vi "Shutter Tuning Interface.vi"(4 "Legacy thrsh (nA)":sgl=0.005 min=0 step=0.0005, 6 "Damped thrsh (nA)":sgl=0.004999995 min=0 step=0.0005, 7 "Shutter Drive":tag="Log/ao0", 10 "Damping":bool=TRUE, 11 "configuration file path":path=path "D:/3D FIB-SEM Files/Jeiss.ini") -> (3 "SEM shutter status":string, 5 "Damping out":bool)   [LabVIEW 2018]
panel:
  out "Specimen I Graph":dbl[](graph)
  in  "Legacy Pulse (ms)":u16=1000
  in  "Pulse Times":u16[][](array[numeric])
  in  "Restore Defaults":bool
  in  "Read from INI":bool
  in  "Write INI":bool
  out "SDev":sgl format="%.4f"
  in  "OPEN-CLOSE":bool
  in  "stop":bool
  # "Pulse Time Fuctions: \n  DeStick, Start, Swing, Brake, Wait, Retain, zeros."
  # "(Close)"
  # "(Open)"
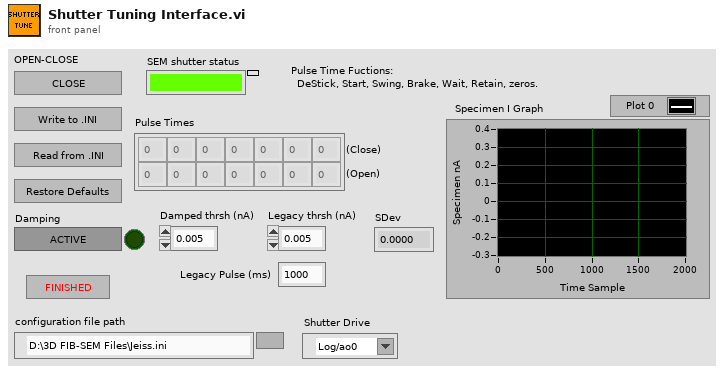
[diagram p1: front panel]
types:
  T1 = cluster{"Legacy thrsh (nA)":sgl, "Damped thrsh (nA)":sgl}
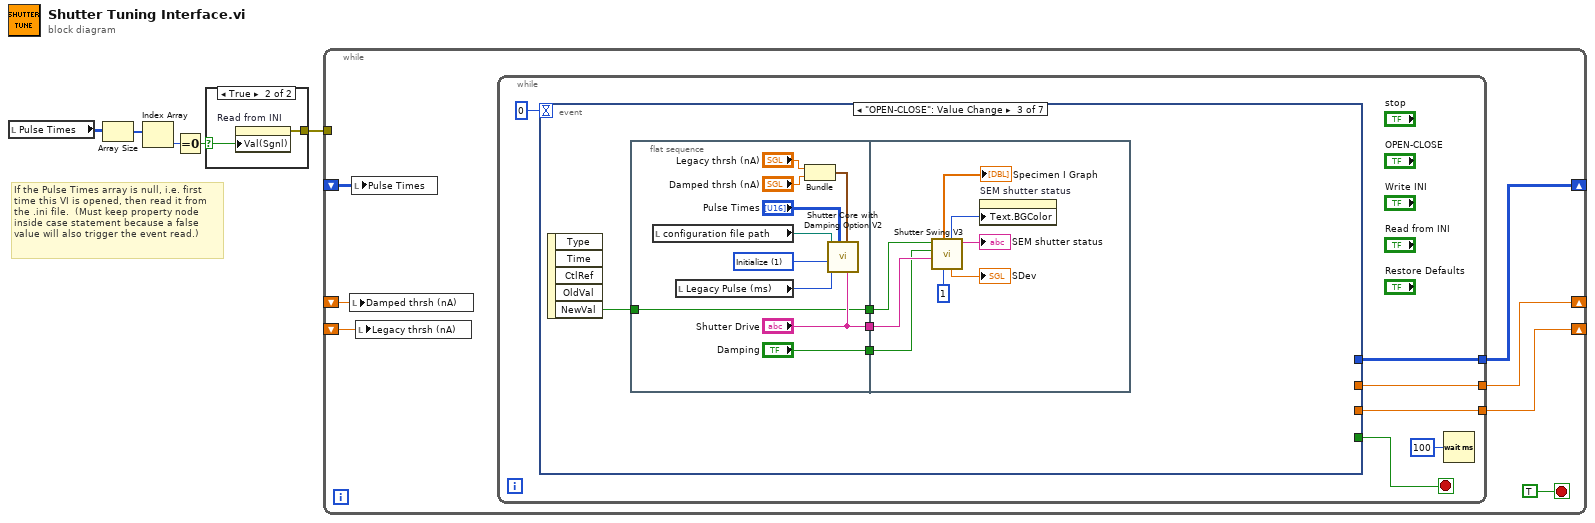
[diagram p0: block diagram]
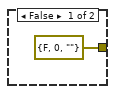
[diagram p2: hidden frame]
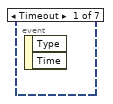
[diagram p3: hidden frame]
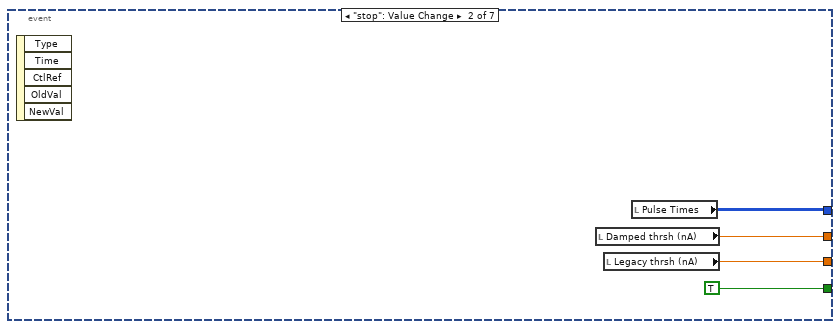
[diagram p4: hidden frame]
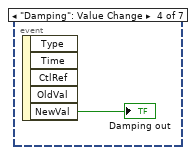
[diagram p5: hidden frame]
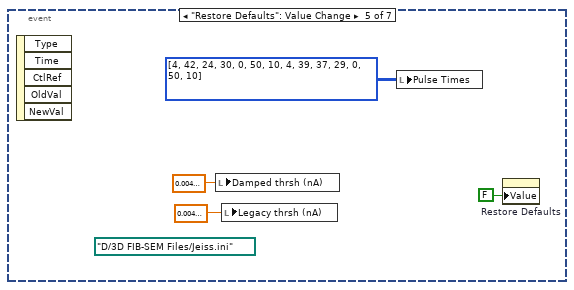
[diagram p6: hidden frame]
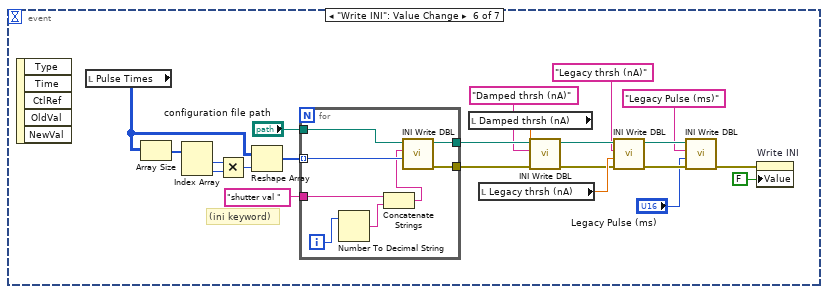
[diagram p7: hidden frame]
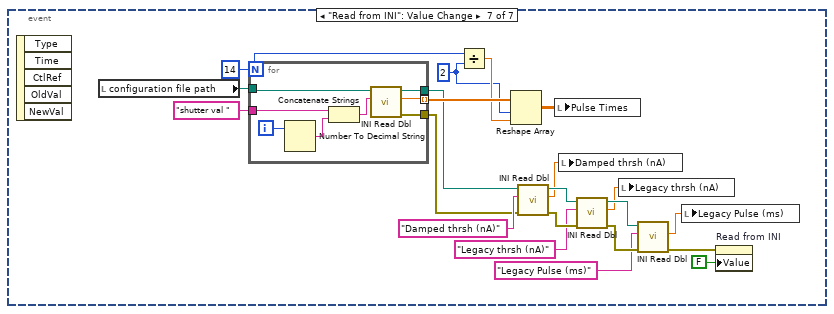
[diagram p8: hidden frame]
diagram:
  # "If the Pulse Times array is null, i.e. first \ntime this VI is opened, then read it from\nthe .ini file.  (Must keep property node\ninside case statement because a false\nvalue will also trigger the event read.)"
  n1 = local read "Pulse Times"() -> (w5:u16[][])
  n2 = Array Size(array=w5) -> (size(s)=w4:i32[])
  n3 = Index Array(array=w4) -> (element=w3:i32)  [unwired: 1 in]
  n4 = Equal To 0?(x=w3) -> (x = 0?=w2:bool)
  n5 = case shown="True" w2 {
    selector: w2 -> [_ w8]
    tunnel: [errorcluster {"status"=FALSE, "code"=0, "source"=""} ("error out") w7] -> w1
    frame False {
    }
    frame True {
      n6 = property on="Read from INI" class="Bool (strict)"("Val(Sgnl)"=w8) -> (error out=w7:errorcluster)  [unwired: 2 in, 1 out]
    }
  }
  n7 = while {
    shift-right: [w10] -> _
    shift-left: _ -> [w9]
    shift-right: [w14] -> _
    shift-left: _ -> [w12]
    shift-right: [w13] -> _
    shift-left: _ -> [w11]
    tunnel: w1 -> [_]
    stop <- TRUE stop-if-true
    n8 = local write "Damped thrsh (nA)"(w12) -> ()
    n9 = local write "Pulse Times"(w9) -> ()
    n10 = local write "Legacy thrsh (nA)"(w11) -> ()
    n11 = while {
      tunnel: [w18] -> w10
      tunnel: [w17] -> w14
      tunnel: [w16] -> w13
      stop <- w19 stop-if-true
      n12 = event shown="[2] \"OPEN-CLOSE\": Value Change" {
        selector: _ -> [_ _ _ _ _ _ _]
        dyn-events: _ -> [_ _ _ _ _ _ _]
        timeout: 0 -> [_ _ _ _ _ _ _]
        tunnel: [_ TRUE _ _ _ _ _] -> w19
        tunnel: [_ w22 _ _ _ _ _] -> w18
        tunnel: [_ w24 _ _ _ _ _] -> w17
        tunnel: [_ w23 _ _ _ _ _] -> w16
        event Timeout {
          n13 = event-data() -> ()  [unwired: 1 in, 2 out]
        }
        event "stop": Value Change {
          n14 = event-data() -> ()  [unwired: 1 in, 5 out]
          n15 = local read "Damped thrsh (nA)"() -> (w24:sgl)
          n16 = local read "Legacy thrsh (nA)"() -> (w23:sgl)
          n17 = local read "Pulse Times"() -> (w22:u16[][])
        }
        event "OPEN-CLOSE": Value Change {
          n18 = event-data() -> ("NewVal"=w27:bool)  [unwired: 1 in, 4 out]
          n19 = flat-sequence {
            tunnel: ["Damping"] -> w29
            tunnel: ["Shutter Drive"] -> w28
            tunnel: w27 -> [w30]
            tunnel: [w30] -> w26
            tunnel: w29 -> [w41]
            tunnel: w28 -> [w42]
            tunnel: w26 -> [w40]
            frame #0 {
              w39 = u16 1 items=["Operate", "Initialize", "Read from .INI", "Write to .INI"] ("Action")
              n20 = local read "configuration file path"() -> (w34:path)
              n21 = local read "Legacy Pulse (ms)"() -> (w33:u16)
              n22 = Bundle("Legacy thrsh (nA)"="Legacy thrsh (nA)", "Damped thrsh (nA)"="Damped thrsh (nA)") -> (w35:T1)  [unwired: 1 in]
              n23 = call "Shutter Core with Damping Option V2.vi"("Shutter Drive"="Shutter Drive", "Thresholds"=w35, "Pulse Times"="Pulse Times", "Legacy Pulse (ms)"=w33, "Action"=w39, "path to .INI file"=w34) -> ()  [unwired: 2 in, 4 out]
            }
            frame #1 {
              n24 = call "Shutter Swing V3.vi"("Retry #"=1, "Shutter Drive"=w42, "Damping"=w41, "Shutter close"=w40) -> ("SEM shutter status"=→"SEM shutter status":string, "SDev"=→"SDev":sgl, "Color Box"=w43:u32, "Specimen I Graph"=→"Specimen I Graph":dbl[])  [unwired: 1 in, 3 out]
              n25 = property on="SEM shutter status" class="Str"("Text.BGColor"=w43) -> ()  [unwired: 2 in, 2 out]
            }
          }
        }
        event "Damping": Value Change {
          n26 = event-data() -> ("NewVal"=→"Damping out":bool)  [unwired: 1 in, 4 out]
        }
        event "Restore Defaults": Value Change {
          (unwired) path "D:/3D FIB-SEM Files/Jeiss.ini" ("path to .INI file")
          n27 = event-data() -> ()  [unwired: 1 in, 5 out]
          n28 = local write "Damped thrsh (nA)"(sgl 0.005 ("Damped thrsh (nA)")) -> ()
          n29 = local write "Legacy thrsh (nA)"(sgl 0.005 ("Damped thrsh (nA)")) -> ()
          n30 = local write "Pulse Times"(u16[][] [[4, 42, 24, 30, 0, 50, 10], [4, 39, 37, 29, 0, 50, 10]] ("Pulse Times")) -> ()
          n31 = property on="Restore Defaults" class="Bool (strict)"("Value"=FALSE ("Restore Defaults")) -> ()  [unwired: 2 in, 2 out]
        }
        event "Write INI": Value Change {
          # "(ini keyword)"
          n32 = event-data() -> ()  [unwired: 1 in, 5 out]
          n33 = local read "Pulse Times"() -> (w57:u16[][])
          n34 = Array Size(array=w57) -> (size(s)=w56:i32[])
          n35 = Index Array(array=w56) -> (element #1=w54:i32, element #2=w55:i32)  [unwired: 2 in]
          n36 = Multiply(x=w54, y=w55) -> (x*y=w53:i32)
          n37 = Reshape Array(w57, w53) -> (w74:u16[])
          n38 = for {
            tunnel: w74 -> [w82] mode=indexing
            tunnel: [w78] -> w73
            tunnel: [w77] -> w67
            tunnel: "configuration file path" -> [w76]
            tunnel: "shutter val " ("Key Str") -> [w75]
            i -> [w81]
            n39 = Number To Decimal String(number=w81) -> (decimal integer string=w80:string)  [unwired: 1 in]
            n40 = Concatenate Strings(w75, w80) -> (w79:string)
            n41 = call "INI Write DBL.vi"("Value In"=w82, "Key Str"=w79, "configuration file path"=w76) -> ("error out"=w77:errorcluster, "file path Out"=w78:path)  [unwired: 7 in]
          }
          n42 = local read "Damped thrsh (nA)"() -> (w71:sgl)
          n43 = local read "Legacy thrsh (nA)"() -> (w68:sgl)
          n44 = call "INI Write DBL.vi"("error IN"=w67, "Value In"=w71, "Key Str"="Damped thrsh (nA)", "configuration file path"=w73) -> ("error out"=w66:errorcluster, "file path Out"=w70:path)  [unwired: 6 in]
          n45 = call "INI Write DBL.vi"("error IN"=w66, "Value In"=w68, "Key Str"="Legacy thrsh (nA)", "configuration file path"=w70) -> ("error out"=w64:errorcluster, "file path Out"=w65:path)  [unwired: 6 in]
          n46 = call "INI Write DBL.vi"("error IN"=w64, "Value In"="Legacy Pulse (ms)", "Key Str"="Legacy Pulse (ms)", "configuration file path"=w65) -> ("error out"=w61:errorcluster)  [unwired: 6 in, 1 out]
          n47 = property on="Write INI" class="Bool (strict)"(error in=w61, "Value"=FALSE ("Write INI")) -> ()  [unwired: 1 in, 2 out]
        }
        event "Read from INI": Value Change {
          w83 = 2 ("y")
          w85 = 14
          n48 = event-data() -> ()  [unwired: 1 in, 5 out]
          n49 = local read "configuration file path"() -> (w103:path)
          n50 = for {
            N: w85 -> [_]
            tunnel: w103 -> [w108]
            tunnel: "shutter val " ("Key Str") -> [w107]
            tunnel: [w106] -> w89
            tunnel: [w105] -> w101 mode=indexing
            tunnel: [w104] -> w88
            i -> [w111]
            n51 = Number To Decimal String(number=w111) -> (decimal integer string=w110:string)  [unwired: 1 in]
            n52 = Concatenate Strings(w107, w110) -> (w109:string)
            n53 = call "INI Read Dbl.vi"("Key Str"=w109, "configuration file path"=w108) -> ("error out"=w104:errorcluster, "Value Out"=w105:dbl, "file path Out"=w106:path)  [unwired: 7 in]
          }
          n54 = Divide(x=w85, y=w83) -> (x/y=w84:dbl)
          n55 = Reshape Array(w101, w83, w84) -> (w100:dbl[][])
          n56 = call "INI Read Dbl.vi"("error IN"=w88, "Key Str"="Damped thrsh (nA)", "configuration file path"=w89) -> ("error out"=w99:errorcluster, "Value Out"=w92:dbl, "file path Out"=w97:path)  [unwired: 6 in]
          n57 = local write "Pulse Times"(w100) -> ()
          n58 = local write "Damped thrsh (nA)"(w92) -> ()
          n59 = call "INI Read Dbl.vi"("error IN"=w99, "Key Str"="Legacy thrsh (nA)", "configuration file path"=w97) -> ("error out"=w98:errorcluster, "Value Out"=w91:dbl, "file path Out"=w96:path)  [unwired: 6 in]
          n60 = local write "Legacy thrsh (nA)"(w91) -> ()
          n61 = call "INI Read Dbl.vi"("error IN"=w98, "Key Str"="Legacy Pulse (ms)", "configuration file path"=w96) -> ("error out"=w87:errorcluster, "Value Out"=w90:dbl)  [unwired: 6 in, 1 out]
          n62 = local write "Legacy Pulse (ms)"(w90) -> ()
          n63 = property on="Read from INI" class="Bool (strict)"(error in=w87, "Value"=FALSE ("Read from INI")) -> ()  [unwired: 1 in, 2 out]
        }
      }
      n64 = Wait (ms)(milliseconds to wait=u32 100) -> ()  [unwired: 1 out]
    }
  }
